vi "PD250 PWM_v2.vi"(8 "error in (no error) 2":errorcluster, 9 "Board Selector":T1, 10 "HMP VISA":refnum<visa-resource-name>="HMP4040_FTS2", 11 "Control Board VISA":refnum<visa-resource-name>="ControlBoard") -> (0 "error out":errorcluster, 2 "Message OUT":string, 3 "Result (bool)":bool)   [LabVIEW 2022 SP3]
uses:
  Serial Board Com/Board Select.ctl
  HMP4000 Communication/HMP4040_ChannelControlAutomatic.ctl
  <vilib>/DAQmx/read.llb/DAQmx Read (Analog 1D Wfm NChan NSamp).vi
  <vilib>/DAQmx/miscellaneous.llb/DAQmx Fill In Error Info.vi
panel:
  out "Duty Cycle VISA Write":string[](array[string])
  out "ControlBoard OUT":refnum<visa-resource-name>
  in  "Message IN":string=" "
  out "Analysis Leg":i32
  out "Waveforms":T2
  out "Active Leg":i32
  out "Result (color)":u32(colorbox)
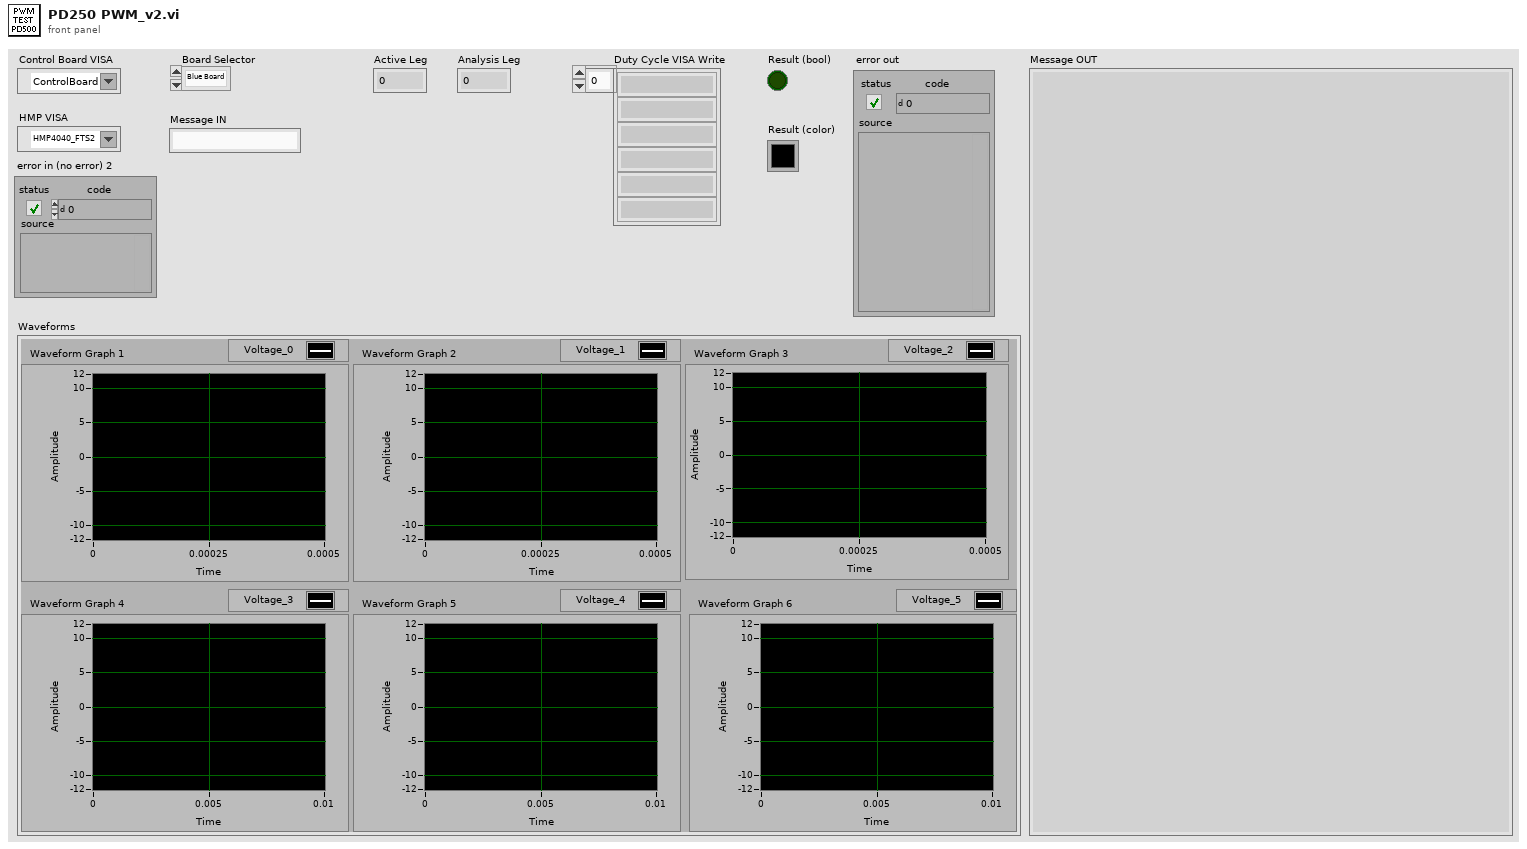
[diagram p1: front panel]
types:
  T1 = typedef "Board Select.ctl" = enum16{"Blue Board", "Green Board"}
  T2 = cluster{"Waveform Graph 1":waveform(dbl), "Waveform Graph 2":waveform(dbl), "Waveform Graph 3":waveform(dbl), "Waveform Graph 4":waveform(dbl), "Waveform Graph 5":waveform(dbl), "Waveform Graph 6":waveform(dbl)}
  T3 = typedef "HMP4040_ChannelControlAutomatic.ctl" = enum16{"Off", "Control Power", "HMP2020 Control + DC32V", "HMP2020 Control + DC8V", "HMP4040 Control + DC32V", "HMP4040 Control +DC8V", "HMP4040 Ch2 24V 4A"}
  T4 = cluster{"data[0]":waveform(dbl), "data[1]":waveform(dbl), "data[2]":waveform(dbl), "data[3]":waveform(dbl), "data[4]":waveform(dbl), "data[5]":waveform(dbl)}
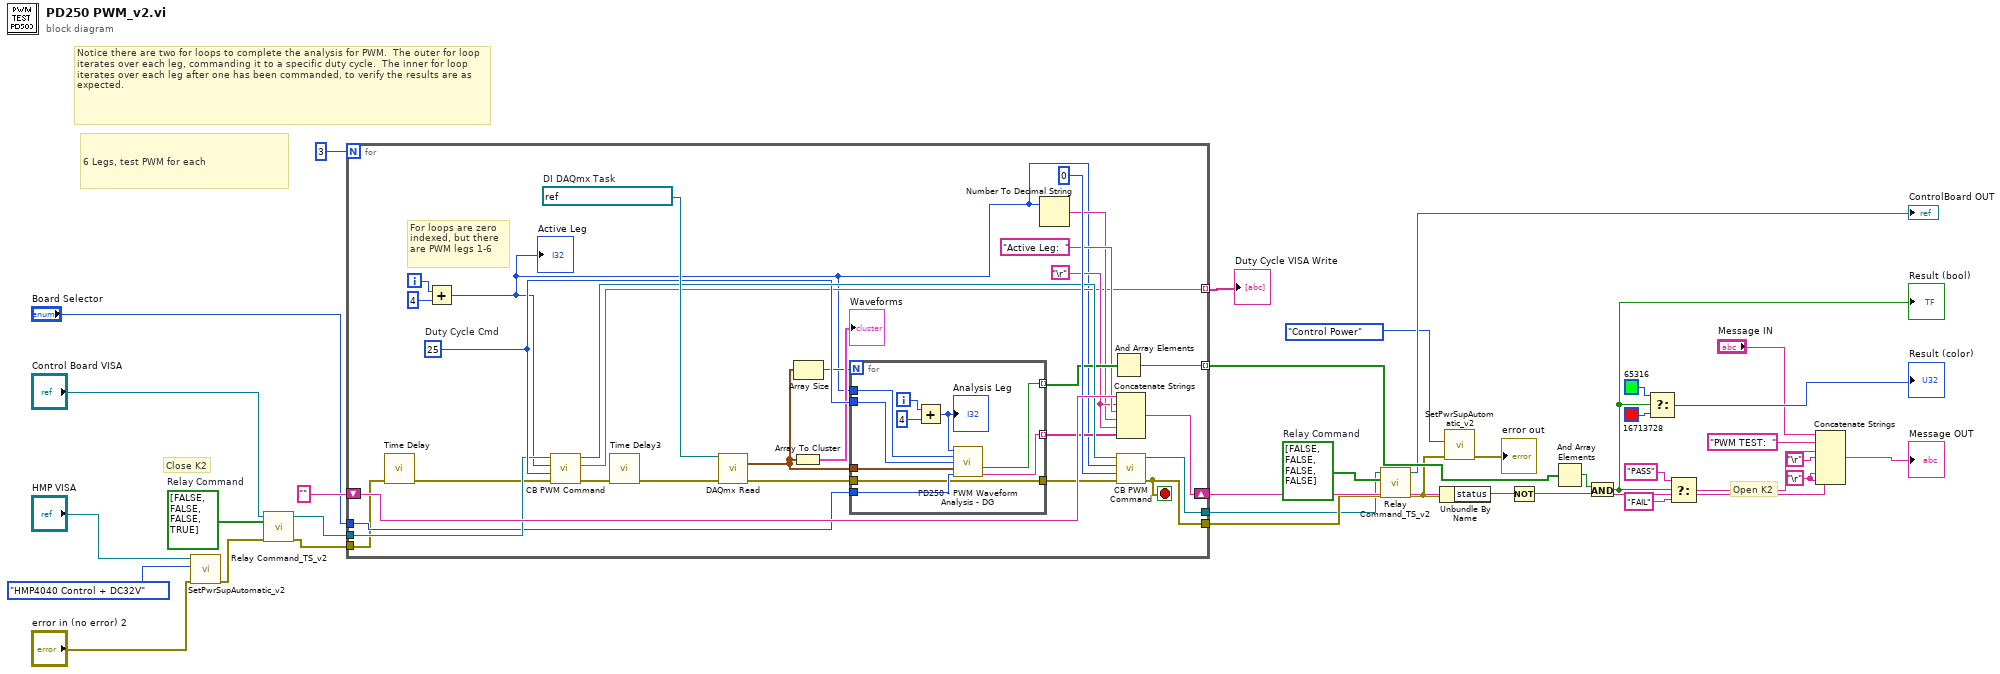
[diagram p0: block diagram]
diagram:
  w12 = bool[] [FALSE, FALSE, FALSE, TRUE]  # Relay Command
  w6 = bool[] [FALSE, FALSE, FALSE, FALSE]  # Relay Command
  w25 = "\r"
  # "Close K2"
  # "Open K2"
  # "Notice there are two for loops to complete the analysis for PWM.  The outer for loop iterates over each leg, commanding it to a specific duty cycle.  The inner for loop iterates over each leg after one has been commanded, to verify the results are as expected."
  # "6 Legs, test PWM for each"
  n1 = call "SetPwrSupAutomatic_v2.vi"("error in (no error)"="error in (no error) 2", "Enum"=HMP4040_ChannelControlAutomatic."HMP4040 Control + DC32V", "HMP VISA"="HMP VISA") -> ("error out"=w10:errorcluster)  [unwired: 7 in, 1 out]
  n2 = call "Relay Command_TS_v2.vi"("error in (no error)"=w10, "Relay Command"=w12, "Control Board VISA"="Control Board VISA") -> ("error out"=w14:errorcluster, "VISA Refnum out"=w15:refnum<visa-resource-name>)  [unwired: 7 in]
  n3 = for {
    N: 3 -> [_]
    tunnel: [w65] -> w36 mode=indexing
    shift-right: [w63] -> w23
    shift-left: "" -> [w62]
    tunnel: [w58] -> w17
    tunnel: [w53] -> w2
    tunnel: w14 -> [w43]
    tunnel: w15 -> [w48]
    tunnel: [w45] -> w13 mode=indexing
    tunnel: "Board Selector" -> [w44]
    i -> [w39]
    stop <- w58 stop-if-true
    w50 = "\r"
    w59 = 25  # Duty Cycle Cmd
    w64 = refnum<k21> "FTS2_PWMInput_DG"  # DI DAQmx Task
    # "For loops are zero indexed, but there are PWM legs 1-6"
    n4 = call "Time Delay"("error in (no error)"=w43) -> ("error out"=w42:errorcluster)  [unwired: 10 in]
    n5 = Add(x=w39, y=4) -> (x+y=w38:i32)
    "Active Leg" <- w38
    n6 = call "CB PWM Command.vi"("error in (no error)"=w42, "Duty Cycle"=w59, "Leg"=w38, "VISA Refnum in"=w48) -> ("error out"=w47:errorcluster, "read buffer"=w45:string, "VISA Refnum out"=w60:refnum<visa-resource-name>)  [unwired: 5 in]
    n7 = call "Time Delay3"("error in (no error)"=w47) -> ("error out"=w46:errorcluster)  [unwired: 10 in]
    n8 = call-poly <vilib>:"DAQmx Read.vi"("task/channels in"=w64, "error in"=w46) -> ("data"=w54:waveform(dbl)[], "error out"=w40:errorcluster)  [unwired: 11 in, 1 out]
    n9 = Array To Cluster(array=w54) -> (cluster=→"Waveforms":T4)
    n10 = Array Size(array=w54) -> (size(s)=w55:i32)
    n11 = for {
      N: w55 -> [_]
      tunnel: w59 -> [w75]
      tunnel: w54 -> [w74]
      tunnel: w38 -> [w73]
      tunnel: [w72] -> w56 mode=indexing
      tunnel: [w71] -> w51 mode=indexing
      tunnel: w44 -> [w70]
      tunnel: [w69] -> w41
      tunnel: w40 -> [w69]
      i -> [w68]
      n12 = Add(x=w68, y=4) -> (x+y=w66:i32)
      "Analysis Leg" <- w66
      n13 = call "PD250 - PWM Waveform Analysis - DG.vi"("Analysis Leg"=w66, "Active Leg"=w73, "Duty Cycle"=w75, "Waveform"=w74, "Board Selector"=w70) -> ("Result (Boolean)"=w72:bool, "Message"=w71:string)  [unwired: 9 in]
    }
    n14 = Number To Decimal String(number=w38) -> (decimal integer string=w49:string)  [unwired: 1 in]
    n15 = And Array Elements(Boolean array=w56) -> (logical AND=w65:bool)
    n16 = Concatenate Strings(w62, w50, "Active Leg:  ", w49, w50, w51) -> (w63:string)
    n17 = call "CB PWM Command.vi"("error in (no error)"=w41, "Duty Cycle"=0, "Leg"=w38, "VISA Refnum in"=w60) -> ("error out"=w58:errorcluster, "VISA Refnum out"=w53:refnum<visa-resource-name>)  [unwired: 5 in, 1 out]
  }
  "Duty Cycle VISA Write" <- w13
  n18 = call "Relay Command_TS_v2.vi"("error in (no error)"=w17, "Relay Command"=w6, "Control Board VISA"=w2) -> ("error out"=w9:errorcluster, "VISA Refnum out"=→"ControlBoard OUT":refnum<visa-resource-name>)  [unwired: 7 in]
  n19 = Unbundle By Name(w9) -> ("status"=w29:bool)
  n20 = call "SetPwrSupAutomatic_v2.vi"("error in (no error)"=w9, "Enum"=HMP4040_ChannelControlAutomatic."Control Power") -> ("error out"=→"error out":errorcluster)  [unwired: 8 in, 1 out]
  n21 = Not(x=w29) -> (.not. x?=w28:bool)
  n22 = And Array Elements(Boolean array=w36) -> (logical AND=w26:bool)
  n23 = And(x=w26, y=w28) -> (x .and. y?=w27:bool)
  "Result (bool)" <- w27
  n24 = Select(t=u32 65316 ("Result (color)"), s=w27, f=u32 16713728 ("Result (color)")) -> (s? t:f=→"Result (color)":u32)
  n25 = Select(t="PASS", s=w27, f="FAIL") -> (s? t:f=w18:string)
  n26 = Concatenate Strings("Message IN", "PWM TEST:  ", w18, "\r", w23, w25, w25) -> (→"Message OUT":string)
